vi "Main.vi"(8 "error in (no error)":errorcluster, 11 "ModuleAdmin":refnum<class "ModuleAdmin.lvclass">) -> ()   [LabVIEW 2014, in "FGenModule.lvlib"]
uses:
  FGenModule.lvlib
  <userlib>/NIST/ModuleAdminLib/ModuleAdmin/ModuleAdmin.lvclass
  PublicAPI/Arguments/Requests/clStopArgument.ctl
  FGenPlugins/MyPluginBaseClass/NISTFGenPluginsBase.lvclass
  <userlib>/NIST/ModuleAdminLib/ModuleAdmin/ModuleAdmin.lvclass/ModuleAdmin.ctl
  FGenPlugins/MyPluginBaseClass/TypeDef/PluginParams.ctl
  <userlib>/NIST/BaseClasses/BasePlugin_class/BasePlugin.lvclass/BasePlugin.ctl
  FGenPlugins/MyPluginBaseClass/TypeDef/OperateModeParams.ctl
  FGenPlugins/MyPluginBaseClass/TypeDef/OutputEnableParams.ctl
  FGenPlugins/MyPluginBaseClass/TypeDef/OutputModeParams.ctl
  FGenPlugins/MyPluginBaseClass/TypeDef/RefClkSourceParams.ctl
  FGenPlugins/MyPluginBaseClass/TypeDef/ChannelNameParams.ctl
  FGenPlugins/MyPluginBaseClass/TypeDef/ConfigStdWaveformParams.ctl
  FGenPlugins/MyPluginBaseClass/TypeDef/ClrArbWfrmParams.ctl
  FGenPlugins/MyPluginBaseClass/TypeDef/CreateArbWfrmParams.ctl
  FGenPlugins/MyPluginBaseClass/TypeDef/ConfigArbWfrmParams.ctl
  FGenPlugins/MyPluginBaseClass/TypeDef/ConfigArbWfrmSRatParams.ctl
  FGenPlugins/MyPluginBaseClass/TypeDef/TriggerParams.ctl
  FGenPlugins/MyPluginBaseClass/TypeDef/ChannelParams.ctl
  FGenPlugins/MyPluginBaseClass/TypeDef/ChannelParamElement.ctl
  FGenPlugins/MyPluginBaseClass/NISTFGenPluginsBase.lvclass/NISTFGenPluginsBase.ctl
  <vilib>/Utility/error.llb/DialogType.ctl
  <userlib>/NIST/ModuleAdminLib/ModuleAdmin/Accessors/Read ShowPanel_.vi
  <userlib>/NIST/BaseClasses/BasePlugin_class/Accessors/Read PluginIniFilePath.vi
  FGenPlugins/MyPluginBaseClass/Accessors/Read Timestamp.vi
  <userlib>/NIST/ModuleAdminLib/ModuleAdmin/Accessors/Write ShowPanel_.vi
  <userlib>/NIST/ModuleAdminLib/ModuleAdmin/Accessors/Read CloneRegRef.vi
  <vilib>/Utility/error.llb/Error Cluster From Error Code.vi
  <vilib>/ErrorRing/Error Ring.xnode
  <userlib>/NIST/ModuleAdminLib/CloneRegistration/CloneRegistration.lvclass
  <userlib>/NIST/ModuleAdminLib/ModuleAdmin.lvlib
panel:
  out "error out":errorcluster
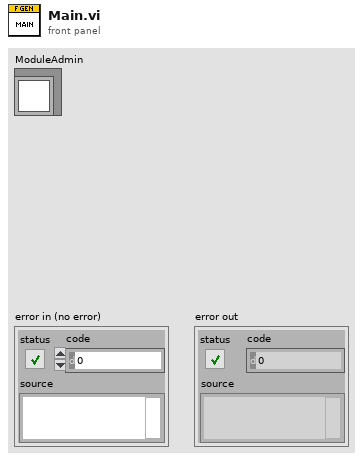
[diagram p1: front panel]
types:
  T1 = typedef "FGenModule.lvlib/clRequestEvents.ctl" = cluster{"StopRequest":refnum<user-event>, "PathToINI":refnum<user-event>, " LoadPlugin":refnum<user-event>, "OperateMode":refnum<user-event>, "OutputEnable":refnum<user-event>, "OutputMode":refnum<user-event>, "RefClkSource":refnum<user-event>, "ChannelName":refnum<user-event>, "Generation":refnum<user-event>, "AbortGeneration":refnum<user-event>, "Reset":refnum<user-event>, "Initialize":refnum<user-event>, "StdWaveform":refnum<user-event>, "ClrArbWfrm":refnum<user-event>, "CreateArbWfrm":refnum<user-event>, "ConfigArbWfrm":refnum<user-event>, "ConfigArbSRat":refnum<user-event>, "GetArbWfrm":refnum<user-event>, "ConfigTriigger":refnum<user-event>, "ShowPanel":refnum<user-event>, "ReadChannelParams":refnum<user-event>, "WriteChannelParams":refnum<user-event>, "ConfigDlg":refnum<user-event>, "Timestamp":refnum<user-event>}
  T2 = typedef "FGenModule.lvlib/clBroadcastEvents.ctl" = cluster{"DidInit":refnum<user-event>, "StatusUpdate":refnum<user-event>, "ErrorReport":refnum<user-event>, "DidStop":refnum<user-event>, "PathToINI":refnum<user-event>, "ChannelName":refnum<user-event>, "ArbWfrmConfig":refnum<user-event>, "ChannelParams":refnum<user-event>, "Timestamp":refnum<user-event>}
  T3 = typedef "FGenModule.lvlib/clStopArgument.ctl" = cluster{"Exit via Stop Module Req?":bool, "Wait for Module to stop?":bool, "ModuleAdmin":refnum<class "ModuleAdmin.lvclass">}
  T4 = enum32{"Invalid", "Standard", "Closed", "Hidden", "Minimized", "Maximized"}
  T5 = typedef "FGenPlugins.lvlib/NISTFGenPluginsBase.lvclass/PluginParams.ctl" = cluster{"Path to Plugin INI":path}
  T6 = typedef "FGenPlugins.lvlib/NISTFGenPluginsBase.lvclass/OperateModeParams.ctl" = cluster{"sName":string, "eOperateMode":u16}
  T7 = typedef "FGenPlugins.lvlib/NISTFGenPluginsBase.lvclass/OutputEnableParams.ctl" = cluster{"sName":string, "bEnabled":bool}
  T8 = typedef "FGenPlugins.lvlib/NISTFGenPluginsBase.lvclass/OutputModeParams.ctl" = cluster{"sName":string, "eOutputMode":u16}
  T9 = typedef "FGenPlugins.lvlib/NISTFGenPluginsBase.lvclass/RefClkSourceParams.ctl" = cluster{"eRefClk":u16}
  T10 = typedef "FGenPlugins.lvlib/NISTFGenPluginsBase.lvclass/ChannelNameParams.ctl" = cluster{"iIndex":i32, "iNameBufferSize":i32}
  T11 = typedef "FGenPlugins.lvlib/NISTFGenPluginsBase.lvclass/ConfigStdWaveformParams.ctl" = cluster{"sName":string, "eWaveform":u16, "dAmplitude":dbl, "dDcOffset":dbl, "dFrequency":dbl, "dStartPhase":dbl, "dSampleRate":dbl, "dNumSamples":dbl}
  T12 = typedef "FGenPlugins.lvlib/NISTFGenPluginsBase.lvclass/ClrArbWfrmParams.ctl" = cluster{"iIndex":i32}
  T13 = typedef "FGenPlugins.lvlib/NISTFGenPluginsBase.lvclass/CreateArbWfrmParams.ctl" = cluster{"sName":string, "iSize":i32, "dData":dbl[], "sWfrmHandle":string}
  T14 = typedef "FGenPlugins.lvlib/NISTFGenPluginsBase.lvclass/ConfigArbWfrmParams.ctl" = cluster{"sName":string, "dGain":dbl, "sWfrmHandle":string, "dOffset":dbl, "dSampleRate":dbl}
  T15 = typedef "FGenPlugins.lvlib/NISTFGenPluginsBase.lvclass/ConfigArbWfrmSRatParams.ctl" = cluster{"sName":string, "dSampleRate":dbl, "sWfrmHandle":string}
  T16 = typedef "FGenPlugins.lvlib/NISTFGenPluginsBase.lvclass/TriggerParams.ctl" = cluster{"eTrigger":u16, "eEdge":u16, "sSource":string}
  T17 = typedef "FGenPlugins.lvlib/NISTFGenPluginsBase.lvclass/ChannelParams.ctl" = T18[]
  T18 = typedef "FGenPlugins.lvlib/NISTFGenPluginsBase.lvclass/ChannelParamElement.ctl" = cluster{"sName":string, "eOperateMode":u16, "bEnabled":bool, "eOutputMode":u16, "iIndex":i32, "iNameBufferSize":i32, "fGain":dbl}
  T19 = typedef "FGenPlugins.lvlib/NISTFGenPluginsBase.lvclass/StdWaveformParams.ctl" = cluster{"eWaveform":u16, "dAmplitude":dbl, "dDcOffset":dbl, "dFrequency":dbl, "dStartPhase":dbl, "dSampleRate":dbl, "dNumSamples":dbl}
  T20 = typedef "FGenPlugins.lvlib/NISTFGenPluginsBase.lvclass/ArbWfrmParams.ctl" = cluster{"sWfrmHandle":string, "iSize":i32, "dData":dbl[], "dGain":dbl, "dOffset":dbl, "dSampleRate":dbl}
  T21 = typedef "NISTFGenPlugins.lvlib/NISTFGenPluginsBase.lvclass/ArbWfrmParams.ctl" = cluster{"sWfrmHandle":string, "iSize":i32, "dData":dbl[], "dGain":dbl, "dOffset":dbl, "dSampleRate":dbl}
  T22 = typedef "DialogType.ctl" = u16
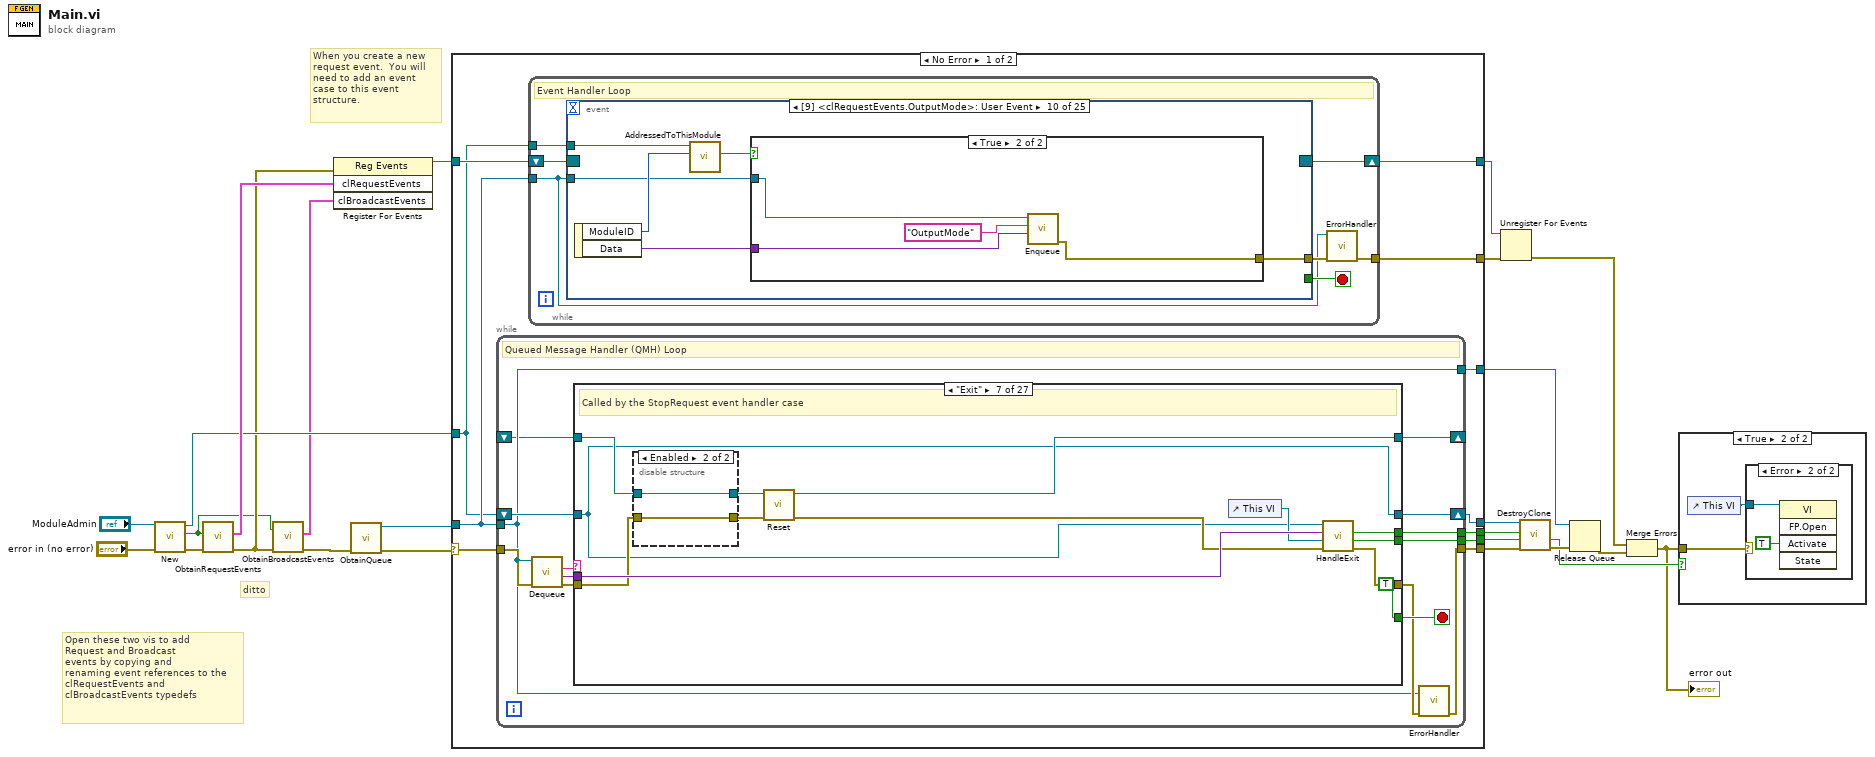
[diagram p0: block diagram]
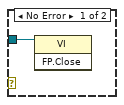
[diagram p3: hidden frame]
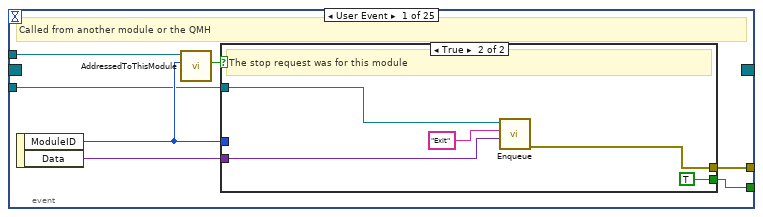
[diagram p4: hidden frame]
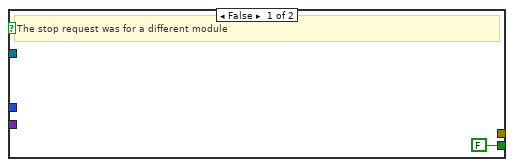
[diagram p5: hidden frame]
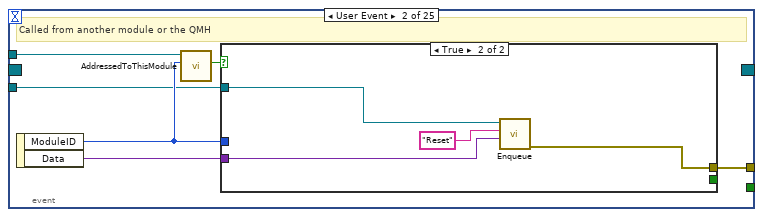
[diagram p6: hidden frame]
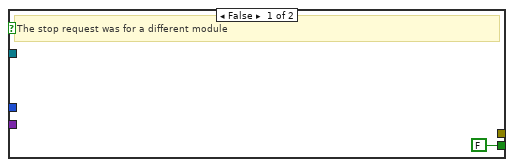
[diagram p7: hidden frame]
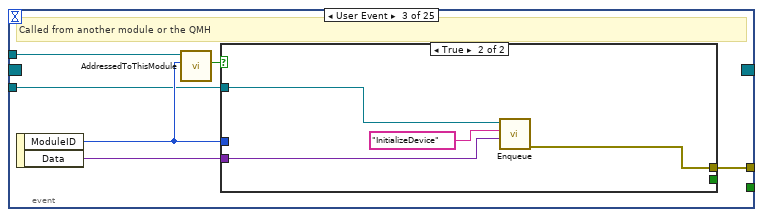
[diagram p8: hidden frame]
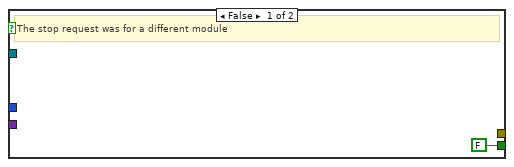
[diagram p9: hidden frame]
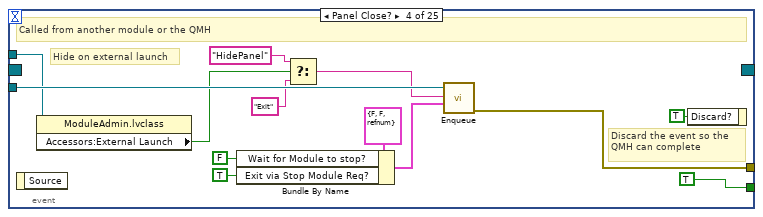
[diagram p10: hidden frame]
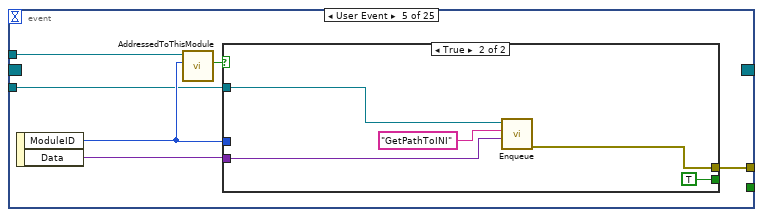
[diagram p11: hidden frame]
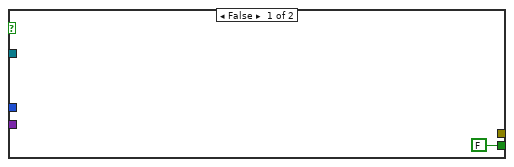
[diagram p12: hidden frame]
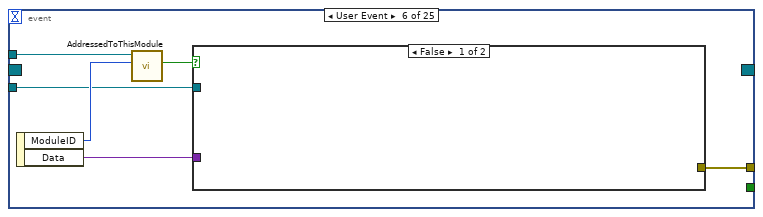
[diagram p13: hidden frame]
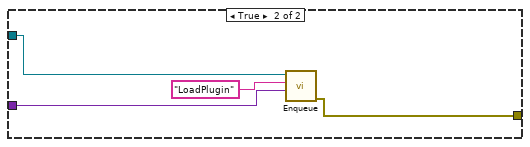
[diagram p14: hidden frame]
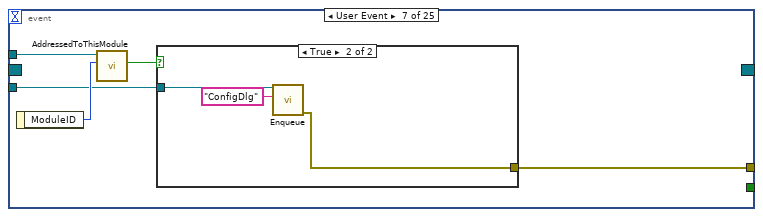
[diagram p15: hidden frame]
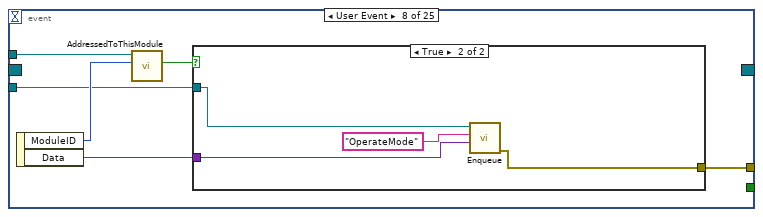
[diagram p17: hidden frame]
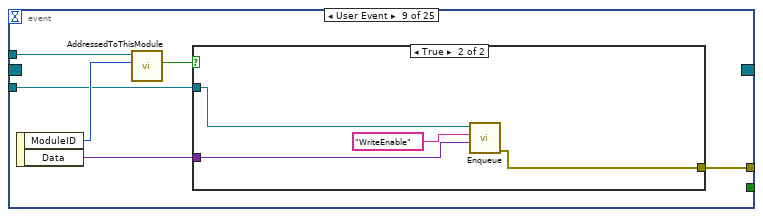
[diagram p19: hidden frame]
diagram:
  # "Open these two vis to add\nRequest and Broadcast \nevents by copying and \nrenaming event references to the \nclRequestEvents and \nclBroadcastEvents typedefs"
  # "ditto"
  # "When you create a new request event.  You will need to add an event case to this event structure."
  n1 = call <userlib>:"New.vi"("error in (no error)"="error in (no error)", "ModuleAdmin"="ModuleAdmin") -> ("error out"=w22:errorcluster, "First?"=w1:bool, "ModuleAdmin"=w18:refnum<class "ModuleAdmin.lvclass">)  [unwired: 7 in]
  n2 = call "ObtainRequestEvents.vi"("error in (no error)"=w22, "CreateNew (f)"=w1) -> ("error out"=w16:errorcluster, "clRequestEvents"=w21:T1)  [unwired: 8 in]
  n3 = call "ObtainBroadcastEvents.vi"("Init? (f)"=w1, "error in (no error)"=w16) -> ("error out"=w6:errorcluster, "clBroadcastEvents"=w15:T2)  [unwired: 8 in]
  n4 = register-events(error in=w16, w21, w15) -> (reference out=w14:refnum<event-registration>)  [unwired: 1 in, 1 out]
  n5 = call "ObtainQueue.vi"("error in (no error)"=w6) -> ("error out"=w20:errorcluster, "MessageQueue"=w19:refnum<queue>)  [unwired: 9 in]
  n6 = case shown="No Error" w20 {
    selector: w20 -> [w35 w832]
    tunnel: w19 -> [w33 w828]
    tunnel: w18 -> [w30 w829]
    tunnel: [w34 w830] -> w13
    tunnel: [w32 w828] -> w17
    tunnel: w14 -> [w31 w824]
    tunnel: [w29 w827] -> w11
    tunnel: [w28 _] -> w10
    tunnel: [w27 _] -> w9
    tunnel: [w26 _] -> w5
    tunnel: [w25 w824] -> w4
    frame No Error {
      n7 = while {
        tunnel: w33 -> [w300]
        tunnel: w35 -> [w309]
        tunnel: [w302] -> w34
        tunnel: [w300] -> w32
        tunnel: [w304] -> w28
        tunnel: [w303] -> w27
        shift-right: [w299] -> _
        shift-left: _ -> [w298]
        shift-right: [w297] -> w29
        shift-left: w30 -> [w305]
        stop <- w310 stop-if-true
        # "Queued Message Handler (QMH) Loop"
        n8 = call "Dequeue.vi"("error in (no error)"=w309, "MessageQueue"=w300) -> ("error out"=w308:errorcluster, "Message Data"=w306:variant, "Message"=w307:string)  [unwired: 6 in, 1 out]
        n9 = case shown="\"Exit\"" w307 {
          selector: w307 -> [w315 _ _ _ _ _ _ _ _ _ _ _ _ _ _ _ _ _ _ _ _ _ _ _ _ _ _]
          tunnel: [_ _ _ _ _ _ TRUE _ _ _ _ _ _ _ _ _ _ _ _ _ _ _ _ _ _ _ _] -> w310
          tunnel: w305 -> [w318 w347 w365 w374 w387 w424 w426 w448 w470 w490 w516 w536 w551 w564 w608 w620 w653 w675 w696 w722 w732 w758 w777 w791 w799 w810 w815]
          tunnel: [w314 w336 w364 w373 w388 w421 w437 w449 w471 w491 w514 w524 w547 w575 w609 w621 w650 w674 w684 w715 w728 w751 w767 w784 w795 w804 w813] -> w301
          tunnel: w308 -> [_ _ w361 w371 w382 w425 w429 w457 w466 w495 w519 w539 w559 w578 w606 w612 w656 w670 w699 w724 w729 w760 w775 w789 w800 w809 w817]
          tunnel: w306 -> [_ _ _ _ w381 _ w436 w456 _ w494 w518 w538 w558 w577 _ _ w657 w671 w700 w725 _ w761 w776 w790 _ _ w818]
          tunnel: [_ _ _ _ _ _ w434 _ _ _ _ _ _ _ _ _ _ _ _ _ _ _ _ _ _ _ _] -> w304
          tunnel: [_ _ _ _ _ _ w433 _ _ _ _ _ _ _ _ _ _ _ _ _ _ _ _ _ _ _ _] -> w303
          tunnel: [w312 refnum<class "NISTFGenPluginsBase.lvclass"> refnum ("MyPlugins.lvlib:MyPluginsBase.lvclass") w360 w370 w385 w422 w432 w447 w467 w492 w498 w534 w552 w566 w610 w622 w649 w672 w685 w712 w726 w748 w768 w779 w792 w803 w812] -> w299
          tunnel: w298 -> [w312 _ w362 w372 w386 w423 w430 w447 w469 w489 w513 w533 w557 w569 w607 w611 w652 w667 w695 w721 w738 w757 w773 w787 w801 w811 w812]
          tunnel: [w311 w331 w359 w369 w375 w424 w426 w446 w464 w482 w509 w525 w548 w563 w605 w619 w636 w661 w682 w703 w727 w741 w765 w782 w793 w802 w814] -> w297
          frame Default {
            # "Called only if a message was queued and no QMH case was created"
            n10 = property class="ModuleAdmin.lvclass"(reference=w318) -> (reference out=w311:refnum<class "ModuleAdmin.lvclass">, "Accessors:Module ID"=w317:i32, "Accessors:ModuleName"=w313:string)  [unwired: 1 in, 1 out]
            n11 = call <userlib>:"ModuleName.vi"("Name"=w313, "ModuleID"=w317) -> ("ModuleName"=w316:string)  [unwired: 9 in]
            n12 = xnode "Error Ring"("parameter 0"=w315, "parameter 1"=w316) -> ("error out"=w314:errorcluster)
          }
          frame "Initialize" {
            # "Initialize is always called after ObtainQueue.vi is run"
            n13 = property class="ModuleAdmin.lvclass"(reference=w347) -> (reference out=w333:refnum<class "ModuleAdmin.lvclass">, error out=w344:errorcluster, "Accessors:Module ID"=w335:i32, "Accessors:ShowPanel_"=w328:bool, "Accessors:External Launch"=w329:bool, "Accessors:ModuleName"=w330:string)  [unwired: 1 in]
            n14 = Compound Arithmetic op=OR(w328, invert w329) -> (w327:bool)
            n15 = Select(t=T4."Standard" ("Front Panel Window:State"), s=w327, f=T4."Hidden" ("Front Panel Window:State")) -> (s? t:f=w340:T4)
            n16 = invoke class="VI" method="FP.Open"(error in=w344, "State"=w340) -> (error out=w343:errorcluster)  [unwired: 3 in, 4 out]
            n17 = call <userlib>:"ModuleName.vi"("Name"=w330, "ModuleID"=w335) -> ("ModuleName"=w339:string)  [unwired: 9 in]
            n18 = property class="VI"(error in=w343, "Front Panel.Title"=w339) -> (reference out=w346:refnum<vi>, error out=w345:errorcluster)  [unwired: 1 in]
            n19 = invoke class="VI" method="FP.Center"(reference=w346, error in=w345) -> (error out=w334:errorcluster)  [unwired: 1 in, 2 out]
            n20 = case shown="True" w329 {
              tunnel: [w348 w354] -> w337
              tunnel: [w349 w351] -> w331
              tunnel: w334 -> [w348 w353]
              tunnel: w333 -> [w349 w350]
              frame False {
              }
              frame True {
                n21 = call <userlib>:"WaitOnModuleSync.vi"("error in (no error)"=w353, "ModuleAdmin"=w350) -> ("error out"=w355:errorcluster, "ModuleAdmin"=w352:refnum<class "ModuleAdmin.lvclass">)  [unwired: 8 in]
                n22 = call <userlib>:"WaitOnEventSync.vi"("error in (no error)"=w355, "ModuleAdmin"=w352) -> ("error out"=w354:errorcluster, "ModuleAdmin"=w351:refnum<class "ModuleAdmin.lvclass">)  [unwired: 8 in]
              }
            }
            n23 = call "DidInit.vi"("Init?"=TRUE, "error in (no error)"=w337, "ModuleAdmin"=w331) -> ("error out"=w336:errorcluster)  [unwired: 8 in]
          }
          frame "Reset" {
            n24 = call-dynamic "Reset.vi"("error in (no error)"=w361, "ClassIn"=w362) -> ("error out"=w357:errorcluster, "ClassOut"=w360:refnum<class "NISTFGenPluginsBase.lvclass">)  [unwired: 8 in]
            n25 = property class="ModuleAdmin.lvclass"(reference=w365, error in=w357) -> (reference out=w359:refnum<class "ModuleAdmin.lvclass">, error out=w356:errorcluster, "Accessors:Module ID"=w363:i32)
            n26 = call "StatusUpdate.vi"("error in (no error)"=w356, "Status"="Device is reset.", "ModuleID"=w363) -> ("error out"=w364:errorcluster)  [unwired: 8 in]
          }
          frame "InitializeDevice" {
            # "Resets device, create channels, sets trigger and clock"
            n27 = property class="ModuleAdmin.lvclass"(reference=w374) -> (reference out=w369:refnum<class "ModuleAdmin.lvclass">, "Accessors:Module ID"=w366:i32)  [unwired: 1 in, 1 out]
            n28 = call-dynamic "Initialize.vi"("error in (no error)"=w371, "ClassIn"=w372) -> ("error out"=w367:errorcluster, "ClassOut"=w370:refnum<class "NISTFGenPluginsBase.lvclass">)  [unwired: 8 in]
            n29 = call "StatusUpdate.vi"("error in (no error)"=w367, "Status"="Device is initialized.", "ModuleID"=w366) -> ("error out"=w373:errorcluster)  [unwired: 8 in]
          }
          frame "LoadPlugin" {
            n30 = Variant To Data(error in=w382, type=T5 {"Path to Plugin INI"=path "../../MyPlugins/Keysight335XX/Keysight335XX.ini"} ("PluginParams"), Variant=w381) -> (data=w384:T5, error out=w380:errorcluster)
            n31 = Unbundle By Name(w384) -> ("Path to Plugin INI"=w377:path)
            n32 = Current VI's Path() -> (path=w378:path)
            n33 = call "GetPluginPath.vi"("error in (no error)"=w380, "Base Path"=w378, "Path to Plugin INI\n(complete)"=w377) -> ("error out"=w379:errorcluster, "Path to Class"=w376:path)  [unwired: 7 in]
            n34 = call <vilib>:"Check if File or Folder Exists.vi"("error in (no error)"=w379, "path"=w376) -> ("error out"=w389:errorcluster, "file or folder exists?"=w391:bool, "dup path"=w390:path)  [unwired: 7 in]
            n35 = case shown="True" w391 {
              tunnel: w390 -> [w395 w413]
              tunnel: w389 -> [_ w412]
              tunnel: [w394 w416] -> w388
              tunnel: w387 -> [w392 w415]
              tunnel: w386 -> [w393 _]
              tunnel: [w393 w410] -> w385
              tunnel: w377 -> [_ w405]
              tunnel: [w392 w404] -> w375
              frame False {
                n36 = Path To String(path=w395) -> (string=w396:string)
                n37 = xnode "Error Ring"("parameter 0"=w396) -> ("error out"=w394:errorcluster)
              }
              frame True {
                # "Initializes the device, sets task, channels, trigger and clock"
                n38 = call-dynamic "LoadClassFromFile.vi"("error in (no error)"=w412, "class path"=w413, "reference in"=refnum<class "NISTFGenPluginsBase.lvclass"> refnum ("MyPlugins.lvlib:MyPluginsBase.lvclass")) -> ("error out"=w407:errorcluster, "reference out"=w408:refnum<class "NISTFGenPluginsBase.lvclass">)  [unwired: 7 in]
                n39 = property class="ModuleAdmin.lvclass"(reference=w415) -> (reference out=w404:refnum<class "ModuleAdmin.lvclass">, "Accessors:Module ID"=w414:i32)  [unwired: 1 in, 1 out]
                n40 = Path To String(path=w413) -> (string=w418:string)
                n41 = call-dynamic "GetDefaultParams.vi"("error in (no error)"=w407, "config file path"=w405, "Class In"=w408) -> ("error out"=w406:errorcluster, "Class Out"=w409:refnum<class "NISTFGenPluginsBase.lvclass">)  [unwired: 7 in]
                n42 = Format Into String(format string="Plugin %s loaded ", w418) -> (resulting string=w417:string)  [unwired: 2 in, 1 out]
                n43 = call "SetDefaultParams.vi"("error in (no error)"=w406, "Class In"=w409) -> ("error out"=w411:errorcluster, "Class Out"=w410:refnum<class "NISTFGenPluginsBase.lvclass">)  [unwired: 8 in]
                n44 = call "StatusUpdate.vi"("error in (no error)"=w411, "Status"=w417, "ModuleID"=w414) -> ("error out"=w416:errorcluster)  [unwired: 8 in]
              }
            }
          }
          frame "ConfigDlg" {
            n45 = call-dynamic "ConfigureDlg.vi"("error in (no error)"=w425, "NISTFGenPluginsBase in"=w423) -> ("error out"=w421:errorcluster, "NISTFGenPluginsBase out"=w422:refnum<class "NISTFGenPluginsBase.lvclass">)  [unwired: 8 in]
          }
          frame "Exit" {
            # "Called by the StopRequest event handler case"
            n46 = disable-structure shown="Enabled" {
              disable-tunnel: w430 -> [w442 w444]
              disable-tunnel: w429 -> [w441 w443]
              disable-tunnel: [w440 w443] -> w428
              disable-tunnel: [w439 w444] -> w427
              frame Disabled {
                n47 = call "DisableAllChannels.vi"("error in (no error)"=w441, "NISTFGenPluginsBase in"=w442) -> ("error out"=w440:errorcluster, "NISTFGenPluginsBase out"=w439:refnum<class "NISTFGenPluginsBase.lvclass">)  [unwired: 8 in]
              }
              frame Enabled {
              }
            }
            n48 = call-dynamic "Reset.vi"("error in (no error)"=w428, "ClassIn"=w427) -> ("error out"=w431:errorcluster, "ClassOut"=w432:refnum<class "NISTFGenPluginsBase.lvclass">)  [unwired: 8 in]
            n49 = control-ref of="This VI"() -> (w435:refnum<vi>)
            n50 = call "HandleExit.vi"("error in (no error)"=w431, "VI Refnum"=w435, "StopArgument"=w436, "ModuleAdmin"=w426) -> ("error out"=w437:errorcluster, "Exit via Stop Module Req?"=w433:bool, "WaitForStop?"=w434:bool)  [unwired: 5 in]
          }
          frame "Error" {
            n51 = property class="ModuleAdmin.lvclass"(reference=w448) -> (reference out=w445:refnum<class "ModuleAdmin.lvclass">, "Accessors:External Launch"=w452:bool, "Accessors:Module ID"=w450:i32)  [unwired: 1 in, 1 out]
            n52 = Variant To Data(error in=w457, type=errorcluster {"status"=FALSE, "code"=0, "source"=""} ("error constant"), Variant=w456) -> (data=w451:errorcluster, error out=w454:errorcluster)
            n53 = call "ReportError.vi"("error in (no error)"=w454, "ErrorReported"=w451, "ModuleID"=w450) -> ("error out"=w453:errorcluster)  [unwired: 8 in]
            n54 = case shown="False" w452 {
              tunnel: w453 -> [w461 w463]
              tunnel: w451 -> [w460 _]
              tunnel: [w459 w463] -> w449
              tunnel: w445 -> [w458 w462]
              tunnel: [w458 w462] -> w446
              frame False {
                # "Todo:  Add an event to ask the user\nIf the module should stop or continue"
                # "Stand alone: now, force an exit"
                n55 = call <vilib>:"Simple Error Handler.vi"("error in (no error)"=w460) -> ()  [unwired: 4 in, 5 out]
                n56 = call "StopRequest.vi"("error in (no error)"=w461, "ModuleAdmin"=w458) -> ("error out"=w459:errorcluster)  [unwired: 8 in, 1 out]
              }
              frame True {
                # "Externally launched modules only broadcast the error msg"
              }
            }
          }
          frame "GetPathToINI" {
            n57 = property class="NISTFGenPluginsBase.lvclass"(reference=w469, error in=w466) -> (reference out=w467:refnum<class "NISTFGenPluginsBase.lvclass">, error out=w465:errorcluster, "Accessors:PluginIniFilePath"=w468:path)
            n58 = property class="ModuleAdmin.lvclass"(reference=w470) -> (reference out=w464:refnum<class "ModuleAdmin.lvclass">, "Accessors:Module ID"=w472:i32)  [unwired: 1 in, 1 out]
            n59 = call "PathToINIBroadcast.vi"("error in (no error)"=w465, "PathToINI"=w468, "ModuleID"=w472) -> ("error out"=w471:errorcluster)  [unwired: 8 in]
          }
          frame "OperateMode" {
            n60 = Variant To Data(error in=w495, type=T6 {"sName"="", "eOperateMode"=0} ("OperateModeParams"), Variant=w494) -> (data=w493:T6, error out=w488:errorcluster)
            n61 = Unbundle By Name(w493) -> ("sName"=w487:string, "eOperateMode"=w479:u16)
            n62 = call "GetChannelIndex.vi"("error in (no error)"=w488, "sName"=w487, "NISTFGenPluginsBase in"=w489) -> ("error out"=w485:errorcluster, "NISTFGenPluginsBase out"=w486:refnum<class "NISTFGenPluginsBase.lvclass">)  [unwired: 7 in]
            n63 = call "StoreOperateMode.vi"("error in (no error)"=w485, "eOperateMode"=w479, "ClassIn"=w486) -> ("error out"=w484:errorcluster, "ClassOut"=w483:refnum<class "NISTFGenPluginsBase.lvclass">)  [unwired: 7 in]
            n64 = call-dynamic "ConfigOperateMode.vi"("error in (no error)"=w484, "ClassIn"=w483) -> ("error out"=w474:errorcluster, "ClassOut"=w492:refnum<class "NISTFGenPluginsBase.lvclass">)  [unwired: 8 in]
            n65 = property class="ModuleAdmin.lvclass"(reference=w490, error in=w474) -> (reference out=w482:refnum<class "ModuleAdmin.lvclass">, error out=w473:errorcluster, "Accessors:Module ID"=w481:i32)
            n66 = Equal?(x=w479, y=u16 1) -> (x = y?=w480:bool)
            n67 = Select(t="Operate Mode is Set to Burst." ("Status"), s=w480, f="Operate Mode is Set to Continuous." ("Status")) -> (s? t:f=w475:string)
            n68 = call "StatusUpdate.vi"("error in (no error)"=w473, "Status"=w475, "ModuleID"=w481) -> ("error out"=w491:errorcluster)  [unwired: 8 in]
          }
          frame "WriteEnable" {
            n69 = Variant To Data(error in=w519, type=T7 {"sName"="", "bEnabled"=FALSE} ("OutputEnableParams"), Variant=w518) -> (data=w517:T7, error out=w512:errorcluster)
            n70 = Unbundle By Name(w517) -> ("sName"=w501:string, "bEnabled"=w507:bool)
            n71 = call "GetChannelIndex.vi"("error in (no error)"=w512, "sName"=w501, "NISTFGenPluginsBase in"=w513) -> ("error out"=w510:errorcluster, "NISTFGenPluginsBase out"=w511:refnum<class "NISTFGenPluginsBase.lvclass">)  [unwired: 7 in]
            n72 = call "StoreOutputEnableMode.vi"("error in (no error)"=w510, "bEnabled"=w507, "ClassIn"=w511) -> ("error out"=w497:errorcluster, "ClassOut"=w498:refnum<class "NISTFGenPluginsBase.lvclass">)  [unwired: 7 in]
            n73 = Select(t="Enabled." ("Status"), s=w507, f="Disabled." ("Status")) -> (s? t:f=w500:string)
            n74 = property class="ModuleAdmin.lvclass"(reference=w516, error in=w497) -> (reference out=w509:refnum<class "ModuleAdmin.lvclass">, error out=w504:errorcluster, "Accessors:Module ID"=w508:i32)
            n75 = Format Into String(format string=" %s %s", initial string="Channel", w501, w500) -> (resulting string=w499:string)  [unwired: 1 in, 1 out]
            n76 = call "StatusUpdate.vi"("error in (no error)"=w504, "Status"=w499, "ModuleID"=w508) -> ("error out"=w514:errorcluster)  [unwired: 8 in]
          }
          frame "OutputMode" {
            n77 = Variant To Data(error in=w539, type=T8 {"sName"="", "eOutputMode"=2} ("OutputModeParams"), Variant=w538) -> (data=w537:T8, error out=w532:errorcluster)
            n78 = Unbundle By Name(w537) -> ("sName"=w531:string, "eOutputMode"=w529:u16)
            n79 = call "GetChannelIndex.vi"("error in (no error)"=w532, "sName"=w531, "NISTFGenPluginsBase in"=w533) -> ("error out"=w528:errorcluster, "NISTFGenPluginsBase out"=w530:refnum<class "NISTFGenPluginsBase.lvclass">)  [unwired: 7 in]
            n80 = call "StoreOutputMode.vi"("error in (no error)"=w528, "eOutputMode"=w529, "ClassIn"=w530) -> ("error out"=w527:errorcluster, "ClassOut"=w526:refnum<class "NISTFGenPluginsBase.lvclass">)  [unwired: 7 in]
            n81 = call-dynamic "ConfigOutputMode.vi"("error in (no error)"=w527, "ClassIn"=w526) -> ("error out"=w520:errorcluster, "ClassOut"=w534:refnum<class "NISTFGenPluginsBase.lvclass">)  [unwired: 8 in]
            n82 = case shown="2" w529 {
              tunnel: ["Ouput Mode Is Set to Function." ("Status") "Ouput Mode is Set to Arbitrary." ("Status") "Ouput Mode is Set to Sequence." ("Status")] -> w523
              frame 0, Default {
              }
              frame 1 {
              }
              frame 2 {
              }
            }
            n83 = property class="ModuleAdmin.lvclass"(reference=w536, error in=w520) -> (reference out=w525:refnum<class "ModuleAdmin.lvclass">, error out=w521:errorcluster, "Accessors:Module ID"=w522:i32)
            n84 = call "StatusUpdate.vi"("error in (no error)"=w521, "Status"=w523, "ModuleID"=w522) -> ("error out"=w524:errorcluster)  [unwired: 8 in]
          }
          frame "RefClkSource" {
            n85 = Variant To Data(error in=w559, type=T9 {"eRefClk"=0} ("RefClkSourceParams"), Variant=w558) -> (data=w556:T9, error out=w554:errorcluster)
            n86 = Unbundle By Name(w556) -> ("eRefClk"=w549:u16)
            n87 = property class="NISTFGenPluginsBase.lvclass"(reference=w557, error in=w554, "Accessors:eRefClk"=w549) -> (reference out=w555:refnum<class "NISTFGenPluginsBase.lvclass">, error out=w553:errorcluster)
            n88 = case shown="0, Default" w549 {
              tunnel: ["Reference Clock Source is Set: Internal." ("Status") "Reference Clock Source is Set: External." ("Status") "Reference Clock Source is Set: RTSI." ("Status")] -> w543
              frame 0, Default {
              }
              frame 1 {
              }
              frame 2 {
              }
            }
            n89 = call-dynamic "ConfigRefClkSource.vi"("error in (no error)"=w553, "ClassIn"=w555) -> ("error out"=w546:errorcluster, "ClassOut"=w552:refnum<class "NISTFGenPluginsBase.lvclass">)  [unwired: 8 in]
            n90 = property class="ModuleAdmin.lvclass"(reference=w551, error in=w546) -> (reference out=w548:refnum<class "ModuleAdmin.lvclass">, error out=w545:errorcluster, "Accessors:Module ID"=w544:i32)
            n91 = call "StatusUpdate.vi"("error in (no error)"=w545, "Status"=w543, "ModuleID"=w544) -> ("error out"=w547:errorcluster)  [unwired: 8 in]
          }
          frame "GetChannelName" {
            n92 = Variant To Data(error in=w578, type=T10 {"iIndex"=0, "iNameBufferSize"=0} ("ChannelNameParams"), Variant=w577) -> (data=w576:T10, error out=w568:errorcluster)
            n93 = Unbundle By Name(w576) -> ("iIndex"=w573:i32, "iNameBufferSize"=w572:i32)
            n94 = call "StoreChannelNameParams.vi"("iNameBufferSize"=w572, "iIndex"=w573, "error in (no error)"=w568, "ClassIn"=w569) -> ("error out"=w571:errorcluster, "ClassOut"=w570:refnum<class "NISTFGenPluginsBase.lvclass">)  [unwired: 6 in]
            n95 = call-dynamic "GetChannelName.vi"("error in (no error)"=w571, "ClassIn"=w570) -> ("error out"=w565:errorcluster, "ClassOut"=w567:refnum<class "NISTFGenPluginsBase.lvclass">)  [unwired: 8 in]
            n96 = case shown="No Error" w565 {
              selector: w565 -> [w588 w595]
              tunnel: [w592 w600] -> w575
              tunnel: w567 -> [w589 w599]
              tunnel: [w587 w599] -> w566
              tunnel: w564 -> [w581 w597]
              tunnel: [w579 w593] -> w563
              frame No Error {
                n97 = property class="NISTFGenPluginsBase.lvclass"(reference=w589, error in=w588) -> (reference out=w587:refnum<class "NISTFGenPluginsBase.lvclass">, error out=w585:errorcluster, "Accessors:ChannelParams"=w591:T18[], "Accessors:iChannelIndex"=w584:i32)
                n98 = property class="ModuleAdmin.lvclass"(reference=w581) -> (reference out=w579:refnum<class "ModuleAdmin.lvclass">, "Accessors:Module ID"=w580:i32)  [unwired: 1 in, 1 out]
                n99 = Index Array(array=w591, index=w584) -> (element=w590:T18)
                n100 = Unbundle By Name(w590) -> ("sName"=w586:string)
                n101 = call "ChannelName.vi"("error in (no error)"=w585, "ChannelName"=w586, "ModuleID"=w580) -> ("error out"=w583:errorcluster)  [unwired: 8 in]
                n102 = call "StatusUpdate.vi"("error in (no error)"=w583, "Status"="Channel Name was Sent.", "ModuleID"=w580) -> ("error out"=w592:errorcluster)  [unwired: 8 in]
              }
              frame Error {
                n103 = property class="ModuleAdmin.lvclass"(reference=w597, error in=w595) -> (reference out=w593:refnum<class "ModuleAdmin.lvclass">, error out=w594:errorcluster, "Accessors:Module ID"=w596:i32)
                n104 = call "ChannelName.vi"("error in (no error)"=w594, "ChannelName"="", "ModuleID"=w596) -> ("error out"=w600:errorcluster)  [unwired: 8 in]
              }
            }
          }
          frame "Generation" {
            n105 = call-dynamic "InitiateGeneration.vi"("error in (no error)"=w606, "ClassIn"=w607) -> ("error out"=w602:errorcluster, "ClassOut"=w610:refnum<class "NISTFGenPluginsBase.lvclass">)  [unwired: 8 in]
            n106 = property class="ModuleAdmin.lvclass"(reference=w608, error in=w602) -> (reference out=w605:refnum<class "ModuleAdmin.lvclass">, error out=w601:errorcluster, "Accessors:Module ID"=w604:i32)
            n107 = call "StatusUpdate.vi"("error in (no error)"=w601, "Status"="Generation Initiated.", "ModuleID"=w604) -> ("error out"=w609:errorcluster)  [unwired: 8 in]
          }
          frame "AbortGeneration" {
            n108 = call "DisableAllChannels.vi"("error in (no error)"=w612, "NISTFGenPluginsBase in"=w611) -> ("error out"=w614:errorcluster, "NISTFGenPluginsBase out"=w613:refnum<class "NISTFGenPluginsBase.lvclass">)  [unwired: 8 in]
            n109 = disable-structure shown="Enabled" {
              disable-tunnel: [w626 w628] -> w622
              disable-tunnel: [w625 w627] -> w616
              disable-tunnel: w614 -> [w624 w627]
              disable-tunnel: w613 -> [w623 w628]
              frame Disabled {
                n110 = call-dynamic "AbortGeneration.vi"("error in (no error)"=w624, "ClassIn"=w623) -> ("error out"=w625:errorcluster, "ClassOut"=w626:refnum<class "NISTFGenPluginsBase.lvclass">)  [unwired: 8 in]
              }
              frame Enabled {
              }
            }
            n111 = property class="ModuleAdmin.lvclass"(reference=w620, error in=w616) -> (reference out=w619:refnum<class "ModuleAdmin.lvclass">, error out=w615:errorcluster, "Accessors:Module ID"=w617:i32)
            n112 = call "StatusUpdate.vi"("error in (no error)"=w615, "Status"="Signal Generation Aborted.", "ModuleID"=w617) -> ("error out"=w621:errorcluster)  [unwired: 8 in]
          }
          frame "StdWaveform" {
            n113 = Variant To Data(error in=w656, type=T11 {"sName"="", "eWaveform"=0, "dAmplitude"=0.1, "dDcOffset"=0.0, "dFrequency"=1000.0, "dStartPhase"=0.0, "dSampleRate"=1000.0, "dNumSamples"=1000.0} ("StdWaveformParams"), Variant=w657) -> (data=w654:T11, error out=w631:errorcluster)
            n114 = property class="NISTFGenPluginsBase.lvclass"(reference=w652, error in=w631) -> (reference out=w632:refnum<class "NISTFGenPluginsBase.lvclass">, error out=w630:errorcluster, "Accessors:StdWaveformParams"=w629:T19)
            n115 = Unbundle By Name(w654) -> ("sName"=w651:string, "eWaveform"=w644:u16, "dAmplitude"=w643:dbl, "dDcOffset"=w642:dbl, "dFrequency"=w641:dbl, "dStartPhase"=w640:dbl, "dSampleRate"=w638:dbl, "dNumSamples"=w637:dbl)
            n116 = Bundle By Name(cluster=w629, "eWaveform"=w644, "dAmplitude"=w643, "dDcOffset"=w642, "dFrequency"=w641, "dStartPhase"=w640, "dSampleRate"=w638, "dNumSamples"=w637) -> (w639:T19)
            n117 = call "GetChannelIndex.vi"("error in (no error)"=w630, "sName"=w651, "NISTFGenPluginsBase in"=w632) -> ("error out"=w646:errorcluster, "NISTFGenPluginsBase out"=w648:refnum<class "NISTFGenPluginsBase.lvclass">)  [unwired: 7 in]
            n118 = property class="NISTFGenPluginsBase.lvclass"(reference=w648, error in=w646, "Accessors:StdWaveformParams"=w639) -> (reference out=w647:refnum<class "NISTFGenPluginsBase.lvclass">, error out=w645:errorcluster)
            n119 = property class="ModuleAdmin.lvclass"(reference=w653) -> (reference out=w636:refnum<class "ModuleAdmin.lvclass">, "Accessors:Module ID"=w634:i32)  [unwired: 1 in, 1 out]
            n120 = call-dynamic "ConfigStdWfrm.vi"("error in (no error)"=w645, "ClassIn"=w647) -> ("error out"=w633:errorcluster, "ClassOut"=w649:refnum<class "NISTFGenPluginsBase.lvclass">)  [unwired: 8 in]
            n121 = call "StatusUpdate.vi"("error in (no error)"=w633, "Status"="Standard Waveform Configured.", "ModuleID"=w634) -> ("error out"=w650:errorcluster)  [unwired: 8 in]
          }
          frame "ClrArbWfrm" {
            n122 = Variant To Data(error in=w670, type=T12 {"iIndex"=0} ("ClrArbWfrmParams"), Variant=w671) -> (data=w668:T12, error out=w666:errorcluster)
            n123 = Unbundle By Name(w668) -> ("iIndex"=w665:i32)
            n124 = Decrement(x=w665) -> (x-1=w662:i32)
            n125 = property class="NISTFGenPluginsBase.lvclass"(reference=w667, error in=w666, "Accessors:iChannelIndex"=w662) -> (reference out=w664:refnum<class "NISTFGenPluginsBase.lvclass">, error out=w663:errorcluster)
            n126 = call-dynamic "ClearArbWfrm.vi"("error in (no error)"=w663, "ClassIn"=w664) -> ("error out"=w660:errorcluster, "ClassOut"=w672:refnum<class "NISTFGenPluginsBase.lvclass">)  [unwired: 8 in]
            n127 = property class="ModuleAdmin.lvclass"(reference=w675, error in=w660) -> (reference out=w661:refnum<class "ModuleAdmin.lvclass">, error out=w659:errorcluster, "Accessors:Module ID"=w673:i32)
            n128 = call "StatusUpdate.vi"("error in (no error)"=w659, "Status"="Arbitrary Waveform was Cleared.", "ModuleID"=w673) -> ("error out"=w674:errorcluster)  [unwired: 8 in]
          }
          frame "CreateArbWfrm" {
            n129 = Variant To Data(error in=w699, type=T13 {"sName"="", "iSize"=0, "dData"=[], "sWfrmHandle"=""} ("CreateArbWfrmParams"), Variant=w700) -> (data=w697:T13, error out=w676:errorcluster)
            n130 = Unbundle By Name(w697) -> ("sName"=w694:string, "iSize"=w691:i32, "dData"=w690:dbl[], "sWfrmHandle"=w689:string)
            n131 = property class="NISTFGenPluginsBase.lvclass"(reference=w695, error in=w676) -> (reference out=w681:refnum<class "NISTFGenPluginsBase.lvclass">, error out=w677:errorcluster, "Accessors:ArbWfrmParams"=w678:T20)
            n132 = Bundle By Name(cluster=w678, "iSize"=w691, "dData"=w690, "sWfrmHandle"=w689) -> (w688:T20)
            n133 = call "GetChannelIndex.vi"("error in (no error)"=w677, "sName"=w694, "NISTFGenPluginsBase in"=w681) -> ("error out"=w692:errorcluster, "NISTFGenPluginsBase out"=w693:refnum<class "NISTFGenPluginsBase.lvclass">)  [unwired: 7 in]
            n134 = property class="NISTFGenPluginsBase.lvclass"(reference=w693, error in=w692, "Accessors:ArbWfrmParams"=w688) -> (reference out=w687:refnum<class "NISTFGenPluginsBase.lvclass">, error out=w686:errorcluster)
            n135 = property class="ModuleAdmin.lvclass"(reference=w696) -> (reference out=w682:refnum<class "ModuleAdmin.lvclass">, "Accessors:Module ID"=w683:i32)  [unwired: 1 in, 1 out]
            n136 = call-dynamic "CreateArbWfrm.vi"("error in (no error)"=w686, "ClassIn"=w687) -> ("error out"=w679:errorcluster, "ClassOut"=w685:refnum<class "NISTFGenPluginsBase.lvclass">)  [unwired: 8 in]
            n137 = call "StatusUpdate.vi"("error in (no error)"=w679, "Status"="Created Arbitrary Waveform", "ModuleID"=w683) -> ("error out"=w684:errorcluster)  [unwired: 8 in]
          }
          frame "ConfigArbWfrm" {
            n138 = Variant To Data(error in=w724, type=T14 {"sName"="", "dGain"=0.0, "sWfrmHandle"="", "dOffset"=0.0, "dSampleRate"=0.0} ("ConfigArbWfrmParams"), Variant=w725) -> (data=w723:T14, error out=w719:errorcluster)
            n139 = Unbundle By Name(w723) -> ("sName"=w720:string, "dOffset"=w718:dbl, "dSampleRate"=w717:dbl, "sWfrmHandle"=w709:string)
            n140 = call "GetChannelIndex.vi"("error in (no error)"=w719, "sName"=w720, "NISTFGenPluginsBase in"=w721) -> ("error out"=w705:errorcluster, "NISTFGenPluginsBase out"=w708:refnum<class "NISTFGenPluginsBase.lvclass">)  [unwired: 7 in]
            n141 = property class="NISTFGenPluginsBase.lvclass"(reference=w708, error in=w705) -> (reference out=w707:refnum<class "NISTFGenPluginsBase.lvclass">, error out=w706:errorcluster, "Accessors:ArbWfrmParams"=w704:T21)
            n142 = Bundle By Name(cluster=w704, "dOffset"=w718, "dSampleRate"=w717, "sWfrmHandle"=w709) -> (w716:T21)
            n143 = property class="NISTFGenPluginsBase.lvclass"(reference=w707, error in=w706, "Accessors:ArbWfrmParams"=w716) -> (reference out=w713:refnum<class "NISTFGenPluginsBase.lvclass">, error out=w711:errorcluster)
            n144 = property class="ModuleAdmin.lvclass"(reference=w722) -> (reference out=w703:refnum<class "ModuleAdmin.lvclass">, "Accessors:Module ID"=w714:i32)  [unwired: 1 in, 1 out]
            n145 = call-dynamic "ConfigArbWfrm.vi"("error in (no error)"=w711, "ClassIn"=w713) -> ("error out"=w702:errorcluster, "ClassOut"=w712:refnum<class "NISTFGenPluginsBase.lvclass">)  [unwired: 8 in]
            n146 = call "StatusUpdate.vi"("error in (no error)"=w702, "Status"="Configured Arbitrary Waveform", "ModuleID"=w714) -> ("error out"=w715:errorcluster)  [unwired: 8 in]
          }
          frame "GetArbWfrmConfig" {
            n147 = property class="NISTFGenPluginsBase.lvclass"(reference=w738) -> (reference out=w726:refnum<class "NISTFGenPluginsBase.lvclass">, "Accessors:ArbWfrmParams"=w737:T20)  [unwired: 1 in, 1 out]
            n148 = property class="ModuleAdmin.lvclass"(reference=w732) -> (reference out=w727:refnum<class "ModuleAdmin.lvclass">, "Accessors:Module ID"=w731:i32)  [unwired: 1 in, 1 out]
            n149 = Unbundle By Name(w737) -> ("dGain"=w735:dbl, "dOffset"=w734:dbl, "dSampleRate"=w733:dbl)
            n150 = Bundle By Name(cluster=T14 {"sName"="", "dGain"=0.0, "sWfrmHandle"="", "dOffset"=0.0, "dSampleRate"=0.0} ("ConfigArbWfrmParams"), "dGain"=w735, "dOffset"=w734, "dSampleRate"=w733) -> (w730:T14)
            n151 = call "ArbWfrmConfig.vi"("error in (no error)"=w729, "ConfigArbWfrmParams"=w730, "ModuleID"=w731) -> ("error out"=w728:errorcluster)  [unwired: 8 in]
          }
          frame "ConfigArbWfrmSRat" {
            n152 = Variant To Data(error in=w760, type=T15 {"sName"="", "dSampleRate"=0.0, "sWfrmHandle"=""} ("ConfigArbWfrmSRatParams"), Variant=w761) -> (data=w759:T15, error out=w755:errorcluster)
            n153 = property class="NISTFGenPluginsBase.lvclass"(reference=w757) -> (reference out=w743:refnum<class "NISTFGenPluginsBase.lvclass">, "Accessors:ArbWfrmParams"=w742:T20)  [unwired: 1 in, 1 out]
            n154 = Unbundle By Name(w759) -> ("sName"=w756:string, "dSampleRate"=w752:dbl, "sWfrmHandle"=w746:string)
            n155 = Bundle By Name(cluster=w742, "dSampleRate"=w752, "sWfrmHandle"=w746) -> (w744:T20)
            n156 = call "GetChannelIndex.vi"("error in (no error)"=w755, "sName"=w756, "NISTFGenPluginsBase in"=w743) -> ("error out"=w753:errorcluster, "NISTFGenPluginsBase out"=w754:refnum<class "NISTFGenPluginsBase.lvclass">)  [unwired: 7 in]
            n157 = property class="NISTFGenPluginsBase.lvclass"(reference=w754, error in=w753, "Accessors:ArbWfrmParams"=w744) -> (reference out=w749:refnum<class "NISTFGenPluginsBase.lvclass">, error out=w745:errorcluster)
            n158 = property class="ModuleAdmin.lvclass"(reference=w758) -> (reference out=w741:refnum<class "ModuleAdmin.lvclass">, "Accessors:Module ID"=w750:i32)  [unwired: 1 in, 1 out]
            n159 = call-dynamic "ConfigArbWfrmSRat.vi"("error in (no error)"=w745, "ClassIn"=w749) -> ("error out"=w740:errorcluster, "ClassOut"=w748:refnum<class "NISTFGenPluginsBase.lvclass">)  [unwired: 8 in]
            n160 = call "StatusUpdate.vi"("error in (no error)"=w740, "Status"="Configured Arbitrary Waveform Sample Rate", "ModuleID"=w750) -> ("error out"=w751:errorcluster)  [unwired: 8 in]
          }
          frame "ConfigTrigger" {
            n161 = Variant To Data(error in=w775, type=T16 {"eTrigger"=0, "eEdge"=10280, "sSource"=""} ("TriggerParams"), Variant=w776) -> (data=w772:T16, error out=w771:errorcluster)
            n162 = property class="NISTFGenPluginsBase.lvclass"(reference=w773, error in=w771, "Accessors:TriggerParams"=w772) -> (reference out=w770:refnum<class "NISTFGenPluginsBase.lvclass">, error out=w769:errorcluster)
            n163 = call-dynamic "ConfigTrigger.vi"("error in (no error)"=w769, "ClassIn"=w770) -> ("error out"=w763:errorcluster, "ClassOut"=w768:refnum<class "NISTFGenPluginsBase.lvclass">)  [unwired: 8 in]
            n164 = property class="ModuleAdmin.lvclass"(reference=w777, error in=w763) -> (reference out=w765:refnum<class "ModuleAdmin.lvclass">, error out=w762:errorcluster, "Accessors:Module ID"=w766:i32)
            n165 = call "StatusUpdate.vi"("error in (no error)"=w762, "Status"="Set Trigger" ("input 3"), "ModuleID"=w766) -> ("error out"=w767:errorcluster)  [unwired: 8 in]
          }
          frame "WriteChannelParams" {
            n166 = Variant To Data(error in=w789, type=T17 [] ("ChannelParams"), Variant=w790) -> (data=w786:T17, error out=w785:errorcluster)
            n167 = property class="NISTFGenPluginsBase.lvclass"(reference=w787, error in=w785, "Accessors:ChannelParams"=w786) -> (reference out=w779:refnum<class "NISTFGenPluginsBase.lvclass">, error out=w778:errorcluster)
            n168 = property class="ModuleAdmin.lvclass"(reference=w791, error in=w778) -> (reference out=w782:refnum<class "ModuleAdmin.lvclass">, error out=w780:errorcluster, "Accessors:Module ID"=w783:i32)
            n169 = call "StatusUpdate.vi"("error in (no error)"=w780, "Status"="Received Channel Params" ("input 3"), "ModuleID"=w783) -> ("error out"=w784:errorcluster)  [unwired: 8 in]
          }
          frame "ReadChannelParams" {
            n170 = property class="NISTFGenPluginsBase.lvclass"(reference=w801) -> (reference out=w792:refnum<class "NISTFGenPluginsBase.lvclass">, "Accessors:ChannelParams"=w798:T18[])  [unwired: 1 in, 1 out]
            n171 = property class="ModuleAdmin.lvclass"(reference=w799) -> (reference out=w793:refnum<class "ModuleAdmin.lvclass">, "Accessors:Module ID"=w797:i32)  [unwired: 1 in, 1 out]
            n172 = call "ChannelParams.vi"("error in (no error)"=w800, "ChannelParams"=w798, "ModuleID"=w797) -> ("error out"=w796:errorcluster)  [unwired: 8 in]
            n173 = call "StatusUpdate.vi"("error in (no error)"=w796, "Status"="Transmitted ChannelParams", "ModuleID"=w797) -> ("error out"=w795:errorcluster)  [unwired: 8 in]
          }
          frame "GetTimestamp" {
            n174 = property class="NISTFGenPluginsBase.lvclass"(reference=w811) -> (reference out=w803:refnum<class "NISTFGenPluginsBase.lvclass">, "Accessors:Timestamp"=w808:dbl)  [unwired: 1 in, 1 out]
            n175 = property class="ModuleAdmin.lvclass"(reference=w810) -> (reference out=w802:refnum<class "ModuleAdmin.lvclass">, "Accessors:Module ID"=w806:i32)  [unwired: 1 in, 1 out]
            n176 = call "Timestamp.vi"("error in (no error)"=w809, "Timestamp"=w808, "ModuleID"=w806) -> ("error out"=w807:errorcluster)  [unwired: 8 in]
            n177 = call "StatusUpdate.vi"("error in (no error)"=w807, "Status"="Timestamp Transmitted", "ModuleID"=w806) -> ("error out"=w804:errorcluster)  [unwired: 8 in]
          }
          frame "ShowPanel" {
            n178 = Variant To Data(error in=w817, type=TRUE, Variant=w818) -> (data=w816:bool, error out=w820:errorcluster)
            n179 = Select(t=T4."Standard" ("Front Panel Window:State"), s=w816, f=T4."Hidden" ("Front Panel Window:State")) -> (s? t:f=w823:T4)
            n180 = property class="VI"(error in=w820, "FP.State"=w823) -> ()  [unwired: 1 in, 2 out]
            n181 = property class="ModuleAdmin.lvclass"(reference=w815, "Accessors:ShowPanel_"=w816) -> (reference out=w814:refnum<class "ModuleAdmin.lvclass">, error out=w813:errorcluster)  [unwired: 1 in]
          }
        }
        n182 = call "ErrorHandler.vi"("error in (no error)"=w301, "MessageQueue"=w300) -> ("error out"=w302:errorcluster)  [unwired: 8 in, 1 out]
      }
      n183 = while {
        tunnel: w33 -> [w36]
        shift-right: [w40] -> w25
        shift-left: w31 -> [w41]
        tunnel: w30 -> [w39]
        tunnel: [w37] -> w26
        stop <- w42 stop-if-true
        # "Event Handler Loop"
        n184 = event shown="[9] <clRequestEvents.OutputMode>: User Event" {
          selector: w41 -> [_ _ _ _ _ _ _ _ _ _ _ _ _ _ _ _ _ _ _ _ _ _ _ _ _]
          dyn-events: [_ _ _ _ _ _ _ _ _ _ _ _ _ _ _ _ _ _ _ _ _ _ _ _ _] -> w40
          timeout: _ -> [_ _ _ _ _ _ _ _ _ _ _ _ _ _ _ _ _ _ _ _ _ _ _ _ _]
          tunnel: w36 -> [w46 w58 w69 w90 w93 w104 w114 w122 w132 w142 w152 w162 w172 w182 w192 w202 w212 w222 w232 w242 w252 w262 w271 w279 w288]
          tunnel: [w45 _ _ TRUE _ _ _ _ _ _ _ _ _ _ _ _ _ _ _ _ _ _ _ _ _] -> w42
          tunnel: w39 -> [w49 w61 w72 w84 w92 w108 w117 w126 w136 w146 w156 w166 w176 w186 w196 w206 w216 w226 w236 w246 w256 w266 w275 w283 w292]
          tunnel: [w44 w57 w68 w88 w91 w105 w113 w123 w133 w143 w153 w163 w173 w183 w193 w203 w213 w223 w233 w243 w253 w263 w272 w280 w287] -> w38
          event User Event {
            # "Called from another module or the QMH"
            n185 = event-data() -> ("ModuleID"=w47:i32, "Data"=w43:variant)  [unwired: 1 in]
            n186 = call <userlib>:"AddressedToThisModule.vi"("ModuleID"=w47, "ModuleAdmin"=w49) -> ("AddressedToThisInstance?"=w48:bool)  [unwired: 8 in, 1 out]
            n187 = case shown="True" w48 {
              tunnel: w47 -> [_ _]
              tunnel: w46 -> [_ w55]
              tunnel: [FALSE TRUE] -> w45
              tunnel: [_ w53] -> w44
              tunnel: w43 -> [_ w51]
              frame False {
                # "The stop request was for a different module"
              }
              frame True {
                # "The stop request was for this module"
                n188 = call "Enqueue.vi"("Message Data"=w51, "Message"="Exit", "MessageQueue"=w55) -> ("error out"=w53:errorcluster)  [unwired: 7 in, 1 out]
              }
            }
          }
          event User Event {
            # "Called from another module or the QMH"
            n189 = event-data() -> ("ModuleID"=w59:i32, "Data"=w56:variant)  [unwired: 1 in]
            n190 = call <userlib>:"AddressedToThisModule.vi"("ModuleID"=w59, "ModuleAdmin"=w61) -> ("AddressedToThisInstance?"=w60:bool)  [unwired: 8 in, 1 out]
            n191 = case shown="True" w60 {
              tunnel: w59 -> [_ _]
              tunnel: w58 -> [_ w66]
              tunnel: [FALSE _] -> _
              tunnel: [_ w65] -> w57
              tunnel: w56 -> [_ w63]
              frame False {
                # "The stop request was for a different module"
              }
              frame True {
                n192 = call "Enqueue.vi"("Message Data"=w63, "Message"="Reset", "MessageQueue"=w66) -> ("error out"=w65:errorcluster)  [unwired: 7 in, 1 out]
              }
            }
          }
          event User Event {
            # "Called from another module or the QMH"
            n193 = event-data() -> ("ModuleID"=w70:i32, "Data"=w67:variant)  [unwired: 1 in]
            n194 = call <userlib>:"AddressedToThisModule.vi"("ModuleID"=w70, "ModuleAdmin"=w72) -> ("AddressedToThisInstance?"=w71:bool)  [unwired: 8 in, 1 out]
            n195 = case shown="True" w71 {
              tunnel: w70 -> [_ _]
              tunnel: w69 -> [_ w77]
              tunnel: [FALSE _] -> _
              tunnel: [_ w76] -> w68
              tunnel: w67 -> [_ w74]
              frame False {
                # "The stop request was for a different module"
              }
              frame True {
                n196 = call "Enqueue.vi"("Message Data"=w74, "Message"="InitializeDevice", "MessageQueue"=w77) -> ("error out"=w76:errorcluster)  [unwired: 7 in, 1 out]
              }
            }
          }
          event Panel Close? {
            # "Hide on external launch"
            # "Discard the event so the QMH can complete"
            # "Called from another module or the QMH"
            n197 = event-data() -> ()  [unwired: 1 in, 1 out]
            n198 = property class="ModuleAdmin.lvclass"(reference=w84) -> ("Accessors:External Launch"=w79:bool)  [unwired: 1 in, 2 out]
            n199 = Bundle By Name(cluster=T3 {"Exit via Stop Module Req?"=FALSE, "Wait for Module to stop?"=FALSE, "ModuleAdmin"=refnum} ("Stop Argument"), "Wait for Module to stop?"=FALSE, "Exit via Stop Module Req?"=TRUE) -> (w85:T3)
            n200 = Select(t="HidePanel", s=w79, f="Exit" ("Message")) -> (s? t:f=w81:string)
            n201 = call "Enqueue.vi"("Message Data"=w85, "Message"=w81, "MessageQueue"=w90) -> ("error out"=w88:errorcluster)  [unwired: 7 in, 1 out]
            n202 = event-data("Discard?"=TRUE) -> ()  [unwired: 1 in, 1 out]
          }
          event User Event {
            n203 = event-data() -> ("ModuleID"=w94:i32, "Data"=w95:variant)  [unwired: 1 in]
            n204 = call <userlib>:"AddressedToThisModule.vi"("ModuleID"=w94, "ModuleAdmin"=w92) -> ("AddressedToThisInstance?"=w96:bool)  [unwired: 8 in, 1 out]
            n205 = case shown="True" w96 {
              tunnel: w94 -> [_ _]
              tunnel: w93 -> [_ w102]
              tunnel: [FALSE TRUE] -> _
              tunnel: [_ w100] -> w91
              tunnel: w95 -> [_ w98]
              frame False {
                # "The stop request was for a different module"
              }
              frame True {
                # "The stop request was for this module"
                n206 = call "Enqueue.vi"("Message Data"=w98, "Message"="GetPathToINI", "MessageQueue"=w102) -> ("error out"=w100:errorcluster)  [unwired: 7 in, 1 out]
              }
            }
          }
          event User Event {
            n207 = event-data() -> ("ModuleID"=w107:i32, "Data"=w103:variant)  [unwired: 1 in]
            n208 = call <userlib>:"AddressedToThisModule.vi"("ModuleID"=w107, "ModuleAdmin"=w108) -> ("AddressedToThisInstance?"=w106:bool)  [unwired: 8 in, 1 out]
            n209 = case shown="False" w106 {
              tunnel: [_ w109] -> w105
              tunnel: w104 -> [_ w112]
              tunnel: w103 -> [_ w110]
              frame False {
              }
              frame True {
                n210 = call "Enqueue.vi"("Message Data"=w110, "Message"="LoadPlugin", "MessageQueue"=w112) -> ("error out"=w109:errorcluster)  [unwired: 7 in, 1 out]
              }
            }
          }
          event User Event {
            n211 = event-data() -> ("ModuleID"=w116:i32)  [unwired: 1 in]
            n212 = call <userlib>:"AddressedToThisModule.vi"("ModuleID"=w116, "ModuleAdmin"=w117) -> ("AddressedToThisInstance?"=w115:bool)  [unwired: 8 in, 1 out]
            n213 = case shown="True" w115 {
              tunnel: w114 -> [_ w120]
              tunnel: [_ w118] -> w113
              frame False {
              }
              frame True {
                n214 = call "Enqueue.vi"("Message"="ConfigDlg", "MessageQueue"=w120) -> ("error out"=w118:errorcluster)  [unwired: 8 in, 1 out]
              }
            }
          }
          event User Event {
            n215 = event-data() -> ("ModuleID"=w125:i32, "Data"=w121:variant)  [unwired: 1 in]
            n216 = call <userlib>:"AddressedToThisModule.vi"("ModuleID"=w125, "ModuleAdmin"=w126) -> ("AddressedToThisInstance?"=w124:bool)  [unwired: 8 in, 1 out]
            n217 = case shown="True" w124 {
              tunnel: [_ w127] -> w123
              tunnel: w122 -> [_ w130]
              tunnel: w121 -> [_ w128]
              frame False {
              }
              frame True {
                n218 = call "Enqueue.vi"("Message Data"=w128, "Message"="OperateMode", "MessageQueue"=w130) -> ("error out"=w127:errorcluster)  [unwired: 7 in, 1 out]
              }
            }
          }
          event User Event {
            n219 = event-data() -> ("ModuleID"=w135:i32, "Data"=w131:variant)  [unwired: 1 in]
            n220 = call <userlib>:"AddressedToThisModule.vi"("ModuleID"=w135, "ModuleAdmin"=w136) -> ("AddressedToThisInstance?"=w134:bool)  [unwired: 8 in, 1 out]
            n221 = case shown="True" w134 {
              tunnel: [_ w137] -> w133
              tunnel: w132 -> [_ w140]
              tunnel: w131 -> [_ w138]
              frame False {
              }
              frame True {
                n222 = call "Enqueue.vi"("Message Data"=w138, "Message"="WriteEnable", "MessageQueue"=w140) -> ("error out"=w137:errorcluster)  [unwired: 7 in, 1 out]
              }
            }
          }
          event User Event {
            n223 = event-data() -> ("ModuleID"=w145:i32, "Data"=w141:variant)  [unwired: 1 in]
            n224 = call <userlib>:"AddressedToThisModule.vi"("ModuleID"=w145, "ModuleAdmin"=w146) -> ("AddressedToThisInstance?"=w144:bool)  [unwired: 8 in, 1 out]
            n225 = case shown="True" w144 {
              tunnel: [_ w147] -> w143
              tunnel: w142 -> [_ w150]
              tunnel: w141 -> [_ w148]
              frame False {
              }
              frame True {
                n226 = call "Enqueue.vi"("Message Data"=w148, "Message"="OutputMode", "MessageQueue"=w150) -> ("error out"=w147:errorcluster)  [unwired: 7 in, 1 out]
              }
            }
          }
          event User Event {
            n227 = event-data() -> ("ModuleID"=w155:i32, "Data"=w151:variant)  [unwired: 1 in]
            n228 = call <userlib>:"AddressedToThisModule.vi"("ModuleID"=w155, "ModuleAdmin"=w156) -> ("AddressedToThisInstance?"=w154:bool)  [unwired: 8 in, 1 out]
            n229 = case shown="True" w154 {
              tunnel: [_ w157] -> w153
              tunnel: w152 -> [_ w160]
              tunnel: w151 -> [_ w158]
              frame False {
              }
              frame True {
                n230 = call "Enqueue.vi"("Message Data"=w158, "Message"="RefClkSource", "MessageQueue"=w160) -> ("error out"=w157:errorcluster)  [unwired: 7 in, 1 out]
              }
            }
          }
          event User Event {
            n231 = event-data() -> ("ModuleID"=w165:i32, "Data"=w161:variant)  [unwired: 1 in]
            n232 = call <userlib>:"AddressedToThisModule.vi"("ModuleID"=w165, "ModuleAdmin"=w166) -> ("AddressedToThisInstance?"=w164:bool)  [unwired: 8 in, 1 out]
            n233 = case shown="True" w164 {
              tunnel: [_ w167] -> w163
              tunnel: w162 -> [_ w170]
              tunnel: w161 -> [_ w168]
              frame False {
              }
              frame True {
                n234 = call "Enqueue.vi"("Message Data"=w168, "Message"="GetChannelName", "MessageQueue"=w170) -> ("error out"=w167:errorcluster)  [unwired: 7 in, 1 out]
              }
            }
          }
          event User Event {
            n235 = event-data() -> ("ModuleID"=w175:i32, "Data"=w171:variant)  [unwired: 1 in]
            n236 = call <userlib>:"AddressedToThisModule.vi"("ModuleID"=w175, "ModuleAdmin"=w176) -> ("AddressedToThisInstance?"=w174:bool)  [unwired: 8 in, 1 out]
            n237 = case shown="True" w174 {
              tunnel: [_ w177] -> w173
              tunnel: w172 -> [_ w180]
              tunnel: w171 -> [_ w178]
              frame False {
              }
              frame True {
                n238 = call "Enqueue.vi"("Message Data"=w178, "Message"="Generation", "MessageQueue"=w180) -> ("error out"=w177:errorcluster)  [unwired: 7 in, 1 out]
              }
            }
          }
          event User Event {
            n239 = event-data() -> ("ModuleID"=w185:i32, "Data"=w181:variant)  [unwired: 1 in]
            n240 = call <userlib>:"AddressedToThisModule.vi"("ModuleID"=w185, "ModuleAdmin"=w186) -> ("AddressedToThisInstance?"=w184:bool)  [unwired: 8 in, 1 out]
            n241 = case shown="True" w184 {
              tunnel: [_ w187] -> w183
              tunnel: w182 -> [_ w190]
              tunnel: w181 -> [_ w188]
              frame False {
              }
              frame True {
                n242 = call "Enqueue.vi"("Message Data"=w188, "Message"="AbortGeneration", "MessageQueue"=w190) -> ("error out"=w187:errorcluster)  [unwired: 7 in, 1 out]
              }
            }
          }
          event User Event {
            n243 = event-data() -> ("ModuleID"=w195:i32, "Data"=w191:variant)  [unwired: 1 in]
            n244 = call <userlib>:"AddressedToThisModule.vi"("ModuleID"=w195, "ModuleAdmin"=w196) -> ("AddressedToThisInstance?"=w194:bool)  [unwired: 8 in, 1 out]
            n245 = case shown="True" w194 {
              tunnel: [_ w197] -> w193
              tunnel: w192 -> [_ w200]
              tunnel: w191 -> [_ w198]
              frame False {
              }
              frame True {
                n246 = call "Enqueue.vi"("Message Data"=w198, "Message"="StdWaveform", "MessageQueue"=w200) -> ("error out"=w197:errorcluster)  [unwired: 7 in, 1 out]
              }
            }
          }
          event User Event {
            n247 = event-data() -> ("ModuleID"=w205:i32, "Data"=w201:variant)  [unwired: 1 in]
            n248 = call <userlib>:"AddressedToThisModule.vi"("ModuleID"=w205, "ModuleAdmin"=w206) -> ("AddressedToThisInstance?"=w204:bool)  [unwired: 8 in, 1 out]
            n249 = case shown="True" w204 {
              tunnel: [_ w207] -> w203
              tunnel: w202 -> [_ w210]
              tunnel: w201 -> [_ w208]
              frame False {
              }
              frame True {
                n250 = call "Enqueue.vi"("Message Data"=w208, "Message"="ClrArbWfrm", "MessageQueue"=w210) -> ("error out"=w207:errorcluster)  [unwired: 7 in, 1 out]
              }
            }
          }
          event User Event {
            n251 = event-data() -> ("ModuleID"=w215:i32, "Data"=w211:variant)  [unwired: 1 in]
            n252 = call <userlib>:"AddressedToThisModule.vi"("ModuleID"=w215, "ModuleAdmin"=w216) -> ("AddressedToThisInstance?"=w214:bool)  [unwired: 8 in, 1 out]
            n253 = case shown="True" w214 {
              tunnel: [_ w217] -> w213
              tunnel: w212 -> [_ w220]
              tunnel: w211 -> [_ w218]
              frame False {
              }
              frame True {
                n254 = call "Enqueue.vi"("Message Data"=w218, "Message"="CreateArbWfrm", "MessageQueue"=w220) -> ("error out"=w217:errorcluster)  [unwired: 7 in, 1 out]
              }
            }
          }
          event User Event {
            n255 = event-data() -> ("ModuleID"=w225:i32, "Data"=w221:variant)  [unwired: 1 in]
            n256 = call <userlib>:"AddressedToThisModule.vi"("ModuleID"=w225, "ModuleAdmin"=w226) -> ("AddressedToThisInstance?"=w224:bool)  [unwired: 8 in, 1 out]
            n257 = case shown="True" w224 {
              tunnel: [_ w227] -> w223
              tunnel: w222 -> [_ w230]
              tunnel: w221 -> [_ w228]
              frame False {
              }
              frame True {
                n258 = call "Enqueue.vi"("Message Data"=w228, "Message"="ConfigArbWfrm", "MessageQueue"=w230) -> ("error out"=w227:errorcluster)  [unwired: 7 in, 1 out]
              }
            }
          }
          event User Event {
            n259 = event-data() -> ("ModuleID"=w235:i32, "Data"=w231:variant)  [unwired: 1 in]
            n260 = call <userlib>:"AddressedToThisModule.vi"("ModuleID"=w235, "ModuleAdmin"=w236) -> ("AddressedToThisInstance?"=w234:bool)  [unwired: 8 in, 1 out]
            n261 = case shown="True" w234 {
              tunnel: [_ w237] -> w233
              tunnel: w232 -> [_ w240]
              tunnel: w231 -> [_ w238]
              frame False {
              }
              frame True {
                n262 = call "Enqueue.vi"("Message Data"=w238, "Message"="GetArbWfrmConfig", "MessageQueue"=w240) -> ("error out"=w237:errorcluster)  [unwired: 7 in, 1 out]
              }
            }
          }
          event User Event {
            n263 = event-data() -> ("ModuleID"=w245:i32, "Data"=w241:variant)  [unwired: 1 in]
            n264 = call <userlib>:"AddressedToThisModule.vi"("ModuleID"=w245, "ModuleAdmin"=w246) -> ("AddressedToThisInstance?"=w244:bool)  [unwired: 8 in, 1 out]
            n265 = case shown="True" w244 {
              tunnel: [_ w247] -> w243
              tunnel: w242 -> [_ w250]
              tunnel: w241 -> [_ w248]
              frame False {
              }
              frame True {
                n266 = call "Enqueue.vi"("Message Data"=w248, "Message"="ConfigArbWfrmSRat", "MessageQueue"=w250) -> ("error out"=w247:errorcluster)  [unwired: 7 in, 1 out]
              }
            }
          }
          event User Event {
            n267 = event-data() -> ("ModuleID"=w255:i32, "Data"=w251:variant)  [unwired: 1 in]
            n268 = call <userlib>:"AddressedToThisModule.vi"("ModuleID"=w255, "ModuleAdmin"=w256) -> ("AddressedToThisInstance?"=w254:bool)  [unwired: 8 in, 1 out]
            n269 = case shown="True" w254 {
              tunnel: [_ w257] -> w253
              tunnel: w252 -> [_ w260]
              tunnel: w251 -> [_ w258]
              frame False {
              }
              frame True {
                n270 = call "Enqueue.vi"("Message Data"=w258, "Message"="ConfigTrigger", "MessageQueue"=w260) -> ("error out"=w257:errorcluster)  [unwired: 7 in, 1 out]
              }
            }
          }
          event User Event {
            n271 = event-data() -> ("ModuleID"=w265:i32, "Data"=w261:variant)  [unwired: 1 in]
            n272 = call <userlib>:"AddressedToThisModule.vi"("ModuleID"=w265, "ModuleAdmin"=w266) -> ("AddressedToThisInstance?"=w264:bool)  [unwired: 8 in, 1 out]
            n273 = case shown="True" w264 {
              tunnel: [_ w267] -> w263
              tunnel: w262 -> [_ w270]
              tunnel: w261 -> [_ w268]
              frame False {
              }
              frame True {
                n274 = call "Enqueue.vi"("Message Data"=w268, "Message"="WriteChannelParams", "MessageQueue"=w270) -> ("error out"=w267:errorcluster)  [unwired: 7 in, 1 out]
              }
            }
          }
          event User Event {
            n275 = event-data() -> ("ModuleID"=w274:i32)  [unwired: 1 in]
            n276 = call <userlib>:"AddressedToThisModule.vi"("ModuleID"=w274, "ModuleAdmin"=w275) -> ("AddressedToThisInstance?"=w273:bool)  [unwired: 8 in, 1 out]
            n277 = case shown="True" w273 {
              tunnel: [_ w276] -> w272
              tunnel: w271 -> [_ w278]
              frame False {
              }
              frame True {
                n278 = call "Enqueue.vi"("Message"="ReadChannelParams", "MessageQueue"=w278) -> ("error out"=w276:errorcluster)  [unwired: 8 in, 1 out]
              }
            }
          }
          event User Event {
            n279 = event-data() -> ("ModuleID"=w282:i32)  [unwired: 1 in]
            n280 = call <userlib>:"AddressedToThisModule.vi"("ModuleID"=w282, "ModuleAdmin"=w283) -> ("AddressedToThisInstance?"=w281:bool)  [unwired: 8 in, 1 out]
            n281 = case shown="True" w281 {
              tunnel: [_ w284] -> w280
              tunnel: w279 -> [_ w286]
              frame False {
              }
              frame True {
                n282 = call "Enqueue.vi"("Message"="GetTimestamp", "MessageQueue"=w286) -> ("error out"=w284:errorcluster)  [unwired: 8 in, 1 out]
              }
            }
          }
          event User Event {
            n283 = event-data() -> ("ModuleID"=w291:i32, "Data"=w289:variant)  [unwired: 1 in]
            n284 = call <userlib>:"AddressedToThisModule.vi"("ModuleID"=w291, "ModuleAdmin"=w292) -> ("AddressedToThisInstance?"=w290:bool)  [unwired: 8 in, 1 out]
            n285 = case shown="True" w290 {
              tunnel: w289 -> [_ w295]
              tunnel: w288 -> [_ w296]
              tunnel: [_ w293] -> w287
              frame False {
              }
              frame True {
                n286 = call "Enqueue.vi"("Message Data"=w295, "Message"="ShowPanel", "MessageQueue"=w296) -> ("error out"=w293:errorcluster)  [unwired: 7 in, 1 out]
              }
            }
          }
        }
        n287 = call "ErrorHandler.vi"("error in (no error)"=w38, "MessageQueue"=w36) -> ("error out"=w37:errorcluster)  [unwired: 8 in, 1 out]
      }
    }
    frame Error {
      n288 = property class="ModuleAdmin.lvclass"(reference=w829) -> (reference out=w827:refnum<class "ModuleAdmin.lvclass">, "Accessors:CloneRegRef"=w826:refnum<data-value>, "Accessors:Module ID"=w825:i32)  [unwired: 1 in, 1 out]
      n289 = call <userlib>:"Remove.vi"("Module ID"=w825, "CloneRegRef"=w826) -> ("error out"=w831:errorcluster)  [unwired: 7 in, 2 out]
      n290 = flat-sequence {
        tunnel: w832 -> [w835]
        tunnel: w831 -> [_]
        tunnel: [w833] -> w830
        frame #0 {
          w834 = T22 2 items=["no dialog", "OK message", "continue or stop message", "OK message + warnings", "continue/stop + warnings"] ("type of dialog (OK msg:1)")
          n291 = call <vilib>:"Simple Error Handler.vi"("type of dialog (OK msg:1)"=w834, "error in (no error)"=w835) -> ("error out"=w833:errorcluster)  [unwired: 3 in, 4 out]
        }
      }
    }
  }
  n292 = Unregister For Events(event registration refnum=w4, error in=w5) -> (error out=w2:errorcluster)
  n293 = call "DestroyClone.vi"("error in (no error)"=w13, "Exit via Stop Module Req?"=w9, "Wait for Module to stop?"=w10, "ModuleAdmin"=w11) -> ("error out"=w12:errorcluster, "External Launch"=w8:bool)  [unwired: 5 in, 1 out]
  n294 = Release Queue(queue=w17, error in (no error)=w12) -> (error out=w7:errorcluster)  [unwired: 1 in, 2 out]
  n295 = Merge Errors(w2, w7) -> (w3:errorcluster)
  "error out" <- w3
  n296 = case shown="True" w8 {
    tunnel: w3 -> [_ w837]
    frame False {
    }
    frame True {
      n297 = control-ref of="This VI"() -> (w836:refnum<vi>)
      n298 = case shown="Error" w837 {
        tunnel: w836 -> [w838 w839]
        frame No Error {
          n299 = invoke class="VI" method="FP.Close"(reference=w838) -> ()  [unwired: 2 in, 3 out]
        }
        frame Error {
          n300 = invoke class="VI" method="FP.Open"(reference=w839, "Activate"=TRUE ("Activate?")) -> ()  [unwired: 3 in, 5 out]
        }
      }
    }
  }
